vi "Bernoulli Noise Waveform.vi"(6 "sampling info":cluster{"Fs":dbl, "#s":dbl}={"Fs"=1000.0, "#s"=1000.0} {"Fs" format="%.2p"}, 7 "reset signal":bool, 8 "error in (no error)":errorcluster, 10 "seed":i32=-1, 11 "one probability":dbl=0.5 format="%0.2f") -> (0 "error out":errorcluster, 3 "signal out":waveform(u8))   [LabVIEW 2020, in "NI_MABase.lvlib"]
doc: "Generates a pseudorandom pattern of ones and zeros, where the probability of generating a one is <B>one probability</B> and the probability of generating a zero is (1-<B>one probability</B>)."
uses:
  NI_MABase.lvlib
  NI_AALBase.lvlib
panel:
  in  "t0":timestamp
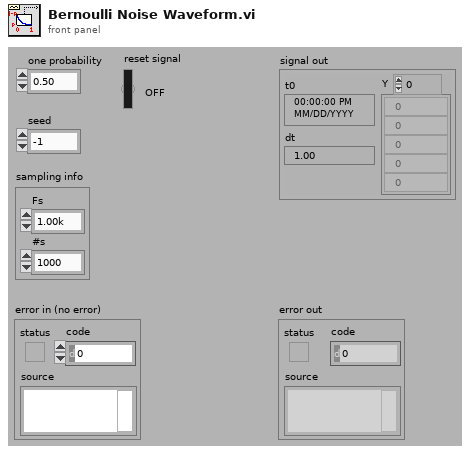
[diagram p1: front panel]
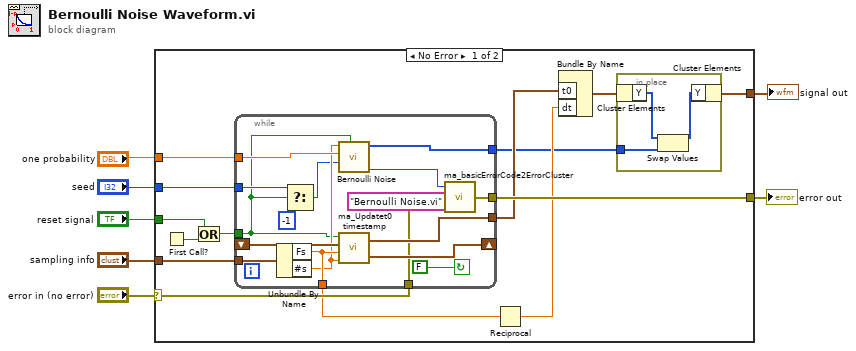
[diagram p0: block diagram]
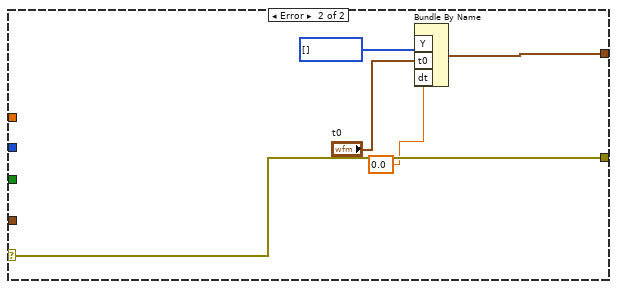
[diagram p2: hidden frame]
diagram:
  n1 = case shown="No Error" "error in (no error)" {
    selector: "error in (no error)" -> [w17 w46]
    tunnel: [w21 w46] -> w7
    tunnel: "sampling info" -> [w20 _]
    tunnel: "one probability" -> [w19 _]
    tunnel: "seed" -> [w18 _]
    tunnel: [w8 w42] -> w2
    tunnel: "reset signal" -> [w11 _]
    frame No Error {
      n2 = First Call?() -> (First Call?: T/F=w13:bool)
      n3 = Or(x=w11, y=w13) -> (x .or. y?=w12:bool)
      n4 = while {
        tunnel: w17 -> [w30]
        tunnel: w12 -> [w25]
        tunnel: w18 -> [w28]
        tunnel: w19 -> [w31]
        tunnel: [w34] -> w16
        tunnel: w20 -> [w35]
        tunnel: [w37] -> w10
        tunnel: [w38] -> w14
        shift-left: _ -> [w40]
        shift-right: [w39] -> _
        tunnel: [w41] -> w21
        stop <- FALSE continue-if-true
        n5 = Unbundle By Name(w35) -> ("Fs"=w34:dbl, "#s"=w29:dbl)
        n6 = Select(t=w28, s=w25, f=-1) -> (s? t:f=w26:i32)
        n7 = call "Bernoulli Noise.vi"("initialize?"=w25, "seed"=w26, "ones probability"=w31, "samples"=w29) -> ("error"=w33:i32, "bernoulli noise"=w37:u8[])  [unwired: 6 in]
        n8 = call "ma_Updatet0 timestamp.vi"("samples"=w29, "sampling rate (S/s)"=w34, "tf previous"=w40, "Reset Generation"=w25) -> ("tf new"=w39:timestamp, "t0"=w38:timestamp)
        n9 = call "ma_basicErrorCode2ErrorCluster.vi"("error in (no error)"=w30, "subVI name"="Bernoulli Noise.vi" ("subVI Name"), "Error Code"=w33) -> ("error out"=w41:errorcluster)
      }
      n10 = Reciprocal(x=w16) -> (1/x=w15:dbl)
      n11 = Bundle By Name("t0"=w14, "dt"=w15) -> (w9:waveform(u8))  [unwired: 1 out]
      n12 = in-place {
        in-place-border: w10 -> [w22]
        n13 = in-place-cluster #1(w9) -> ("Y"=w24:u8[])
        n14 = Swap Values(12:w24, 14:w22) -> (1:w23:u8[])  [unwired: 1 in, 1 out]
        n15 = in-place-cluster #1("Y"=w23) -> (w8:waveform(u8))
      }
    }
    frame Error {
      n16 = Bundle By Name("Y"=u8[] [], "t0"="t0", "dt"=0.0 ("t0")) -> (w42:waveform(u8))  [unwired: 1 out]
    }
  }
  "error out" <- w7
  "signal out" <- w2
